vi "215.XYpos (SubVI).vi"(0 "VISA resource name":refnum<visa-resource-name>="COM7", 7 "X":i32=50 min=0 max=1200 step=1, 9 "Y":i32=50 min=0 max=1200 step=1, 11 "error in (no error)":errorcluster) -> (4 "VISA Out":refnum<visa-resource-name>, 6 "Connected":bool, 8 "Receive string":string, 15 "error out":errorcluster)   [LabVIEW 2017]
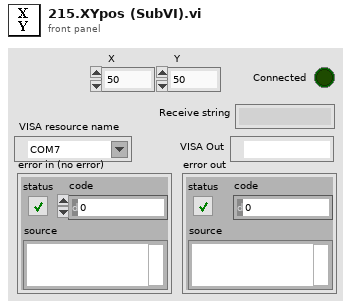
[diagram p1: front panel]
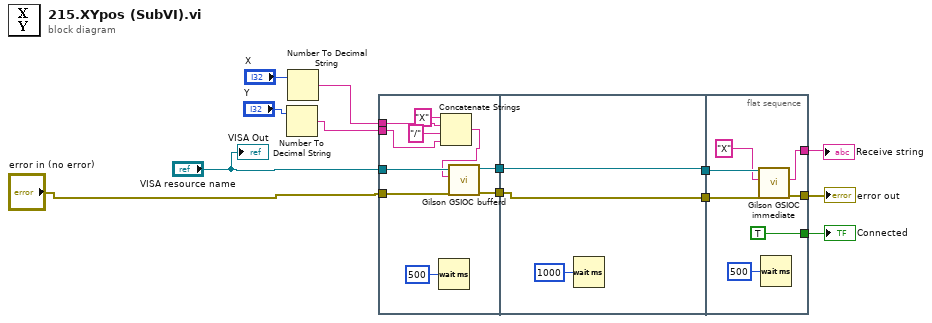
[diagram p0: block diagram]
diagram:
  n1 = Number To Decimal String(number="Y") -> (decimal integer string=w3:string)  [unwired: 1 in]
  n2 = Number To Decimal String(number="X") -> (decimal integer string=w6:string)  [unwired: 1 in]
  n3 = flat-sequence {
    tunnel: "error in (no error)" -> [w23]
    tunnel: "VISA resource name" -> [w21]
    tunnel: [w22] -> w12
    tunnel: [w20] -> w13
    tunnel: w6 -> [w16]
    tunnel: w3 -> [w14]
    tunnel: [w25] -> w11
    tunnel: [w24] -> w10
    tunnel: w13 -> [w25]
    tunnel: w12 -> [w24]
    tunnel: [TRUE] -> w9
    tunnel: w11 -> [w32]
    tunnel: w10 -> [w31]
    tunnel: [w29] -> w8
    tunnel: [w27] -> w7
    frame #0 {
      n4 = Wait (ms)(milliseconds to wait=u32 500) -> ()  [unwired: 1 out]
      n5 = Concatenate Strings("X" ("string"), w16, "/" ("string"), w14) -> (w17:string)
      n6 = call <instrlib>:"Gilson GSIOC bufferd.vi"("error in (no error)"=w23, "Bufferd command"=w17, "VISA resource name"=w21) -> ("error out"=w22:errorcluster, "VISA resource name out"=w20:refnum<visa-resource-name>)  [unwired: 6 in, 1 out]
    }
    frame #1 {
      n7 = Wait (ms)(milliseconds to wait=u32 1000) -> ()  [unwired: 1 out]
    }
    frame #2 {
      n8 = call <instrlib>:"Gilson GSIOC immediate.vi"("error in (no error)"=w31, "Immediate command"="X", "VISA resource name"=w32) -> ("error out"=w29:errorcluster, "Receive string"=w27:string)  [unwired: 6 in, 1 out]
      n9 = Wait (ms)(milliseconds to wait=u32 500) -> ()  [unwired: 1 out]
    }
  }
  "error out" <- w8
  "Connected" <- w9
  "VISA Out" <- "VISA resource name"
  "Receive string" <- w7
